vi "test timestamp from le bytes.vi"(8 "error in (no error)":errorcluster, 11 "TestCase in":refnum<class "Timestamp Tests.lvclass">) -> (0 "error out":errorcluster, 3 "TestCase out":refnum<class "Timestamp Tests.lvclass">)   [LabVIEW 2020, in "Timestamp Tests.lvclass"]
uses:
  Timestamp Tests.lvclass
  <vilib>/addons/_JKI Toolkits/VI Tester/TestCase.llb/TestCase.lvclass
  target/release/labview_test_library.dll
  C:/Program Files/National Instruments/LabVIEW 2020/vi.lib/addons/_JKI Toolkits/VI Tester/TestCase.llb/TestCase.lvclass
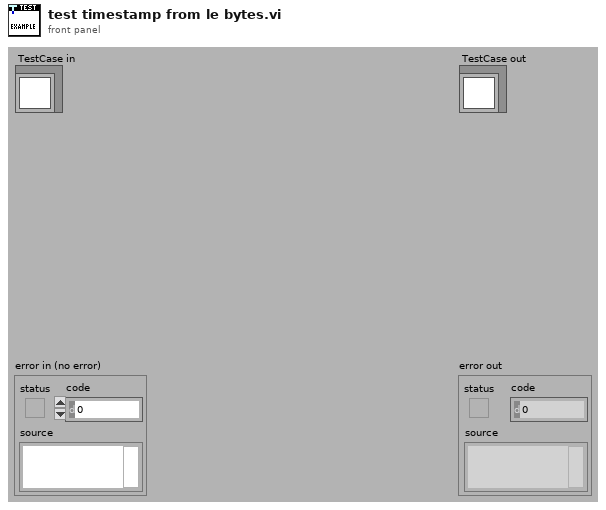
[diagram p1: front panel]
types:
  T1 = enum16{"big-endian, network order", "native, host order", "little-endian"}
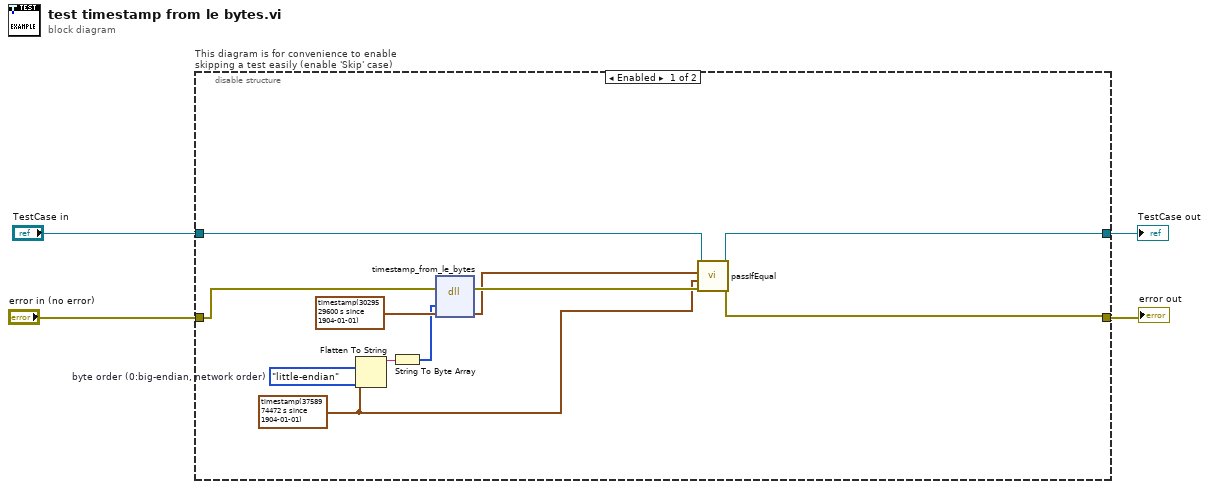
[diagram p0: block diagram]
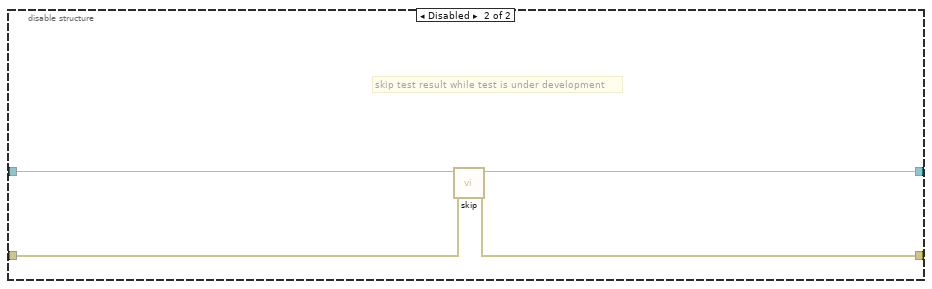
[diagram p2: hidden frame]
diagram:
  n1 = disable-structure "This diagram is for convenience to enable skipping a test easily (enable 'Skip' case)" shown="Enabled" {
    disable-tunnel: "TestCase in" -> [w15 w19]
    disable-tunnel: [w14 w17] -> w1
    disable-tunnel: [w13 w18] -> w3
    disable-tunnel: "error in (no error)" -> [w12 w16]
    frame Enabled {
      w5 = T1."little-endian"  # byte order (0:big-endian, network order)
      w8 = timestamp(3758974472.02441 s since 1904-01-01) ("Time Stamp")
      n2 = Flatten To String(anything=w8, byte order (0:big-endian, network order)=w5) -> (data string=w7:string)  [unwired: 2 in, 2 out]
      n3 = String To Byte Array(string=w7) -> (unsigned byte array=w6:u8[])
      n4 = dll-call lib="C:/Users/JamesMcNally/Documents/RustInterop/Rust-LabVIEW-Interop/target/release/labview_test_library.dll" fn="timestamp_from_le_bytes"(error in=w12, "bytes"=w6, "timestamp"=timestamp(3029529600 s since 1904-01-01) ("Time Stamp")) -> (error out=w11:errorcluster, "timestamp"=w9:timestamp)  [unwired: 4 in, 1 out]
      n5 = call-dynamic "passIfEqual.vi"("error in (no error)"=w11, "y"=w8, "x"=w9, "TestCase in"=w15) -> ("error out"=w13:errorcluster, "TestCase out"=w14:refnum<class "Timestamp Tests.lvclass">)  [unwired: 6 in]
    }
    frame Disabled {
      # "skip test result while test is under development"
      n6 = call <vilib>:"skip.vi"("error in (no error)"=w16, "TestCase in"=w19) -> ("error out"=w18:errorcluster, "TestCase out"=w17:refnum<class "Timestamp Tests.lvclass">)  [unwired: 8 in]
    }
  }
  "error out" <- w3
  "TestCase out" <- w1
